vi "Popup - Splash Screen.vi"(8 "errorIn":errorcluster) -> (0 "errorOut":errorcluster, 3 "Exit":bool)   [LabVIEW 2018, in "Controller (Host).lvlib"]
uses:
  Controller (Host).lvlib
  Globals/Host Globals.vi
panel:
  in  "EXIT":bool
  # "Waiting for cRIO to connect...."
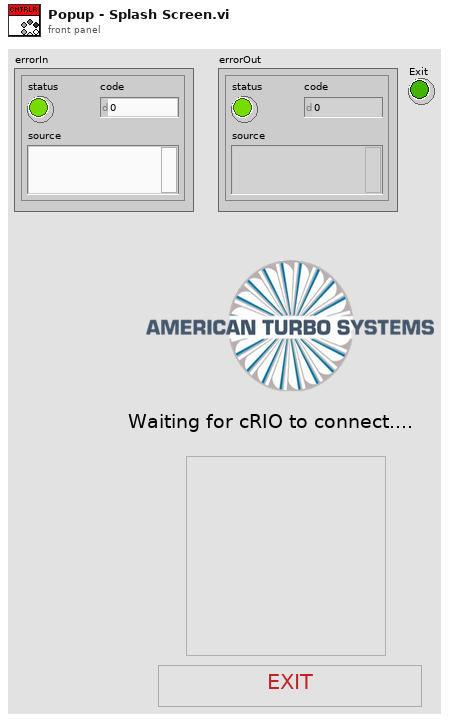
[diagram p1: front panel]
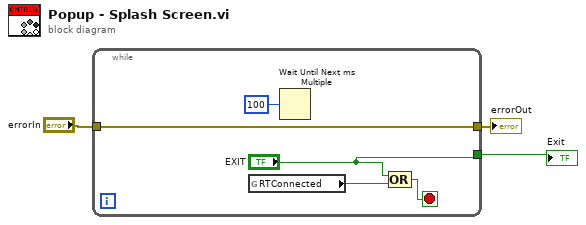
[diagram p0: block diagram]
diagram:
  n1 = while {
    tunnel: "errorIn" -> [w6]
    tunnel: [w6] -> w3
    tunnel: ["EXIT"] -> w2
    stop <- w7 stop-if-true
    n2 = global read "Host Globals.vi" "RTConnected"() -> (w5:bool)
    n3 = Wait Until Next ms Multiple(millisecond multiple=u32 100) -> ()  [unwired: 1 out]
    n4 = Compound Arithmetic op=OR("EXIT", w5) -> (w7:bool)
  }
  "errorOut" <- w3
  "Exit" <- w2
